vi "Make Promise.vi"(8 "error in (no error)":errorcluster, 9 "create if not found? (T)":bool=TRUE, 11 "name (unnamed)":string) -> (0 "error out":errorcluster, 1 "created new?":bool, 3 "Promise out":refnum<class "Promise.lvclass">)   [LabVIEW 2017, in "Promise.lvlib" / "Promise.lvclass"]
doc: "Creates a new promise with an unknown value."
uses:
  Promise.lvclass
panel:
  in  "element data type":variant
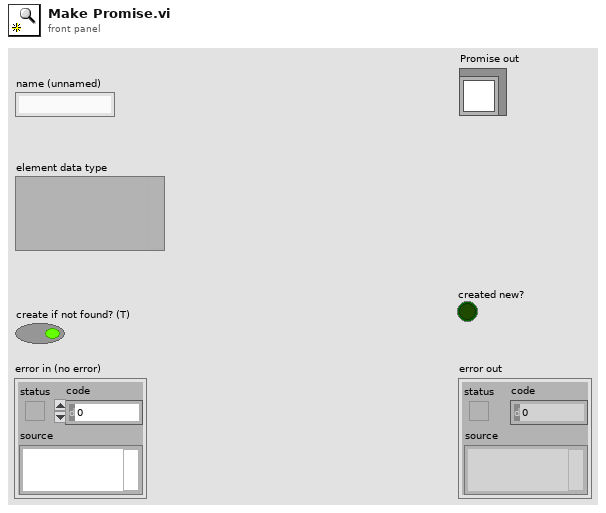
[diagram p1: front panel]
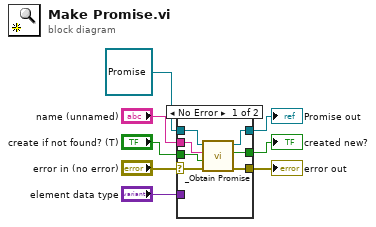
[diagram p0: block diagram]
diagram:
  n1 = case shown="No Error" "error in (no error)" {
    selector: "error in (no error)" -> [w11 w17]
    tunnel: [w15 w17] -> w7
    tunnel: [w13 w16] -> w3
    tunnel: "name (unnamed)" -> [w12 _]
    tunnel: "element data type" -> [_ _]
    tunnel: "create if not found? (T)" -> [w9 _]
    tunnel: refnum<class "Promise.lvclass"> refnum ("Future in") -> [w14 w16]
    tunnel: [w10 _] -> w1
    frame No Error {
      n2 = call-dynamic "_Obtain Promise.vi"("error in (no error)"=w11, "create if not found? (T)"=w9, "name (unnamed)"=w12, "Future in"=w14) -> ("error out"=w15:errorcluster, "created new?"=w10:bool, "Future out"=w13:refnum<class "Promise.lvclass">)  [unwired: 5 in]
    }
    frame Error {
    }
  }
  "error out" <- w7
  "Promise out" <- w3
  "created new?" <- w1
